vi "Main_Source.vi"() -> ()   [LabVIEW 2014]
panel:
  in  "Stop Button":bool
  out "error out":errorcluster
  in  "error in (no error)":errorcluster
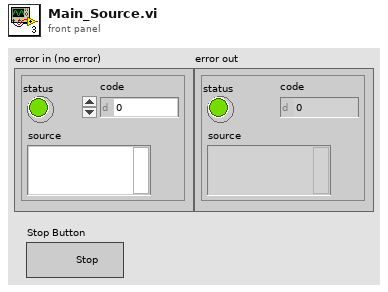
[diagram p1: front panel]
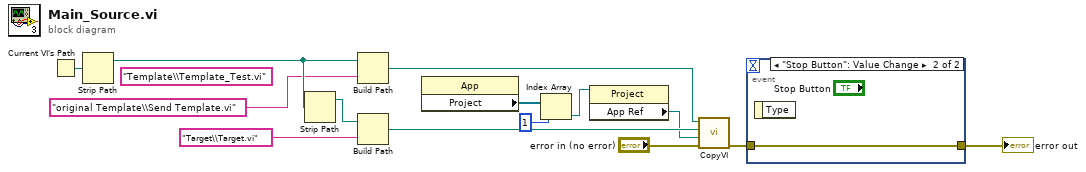
[diagram p0: block diagram]
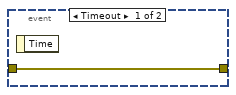
[diagram p2: hidden frame]
diagram:
  (unwired) "Template\\Template_Test.vi" ("name or relative path")
  n1 = Current VI's Path() -> (path=w13:path)
  n2 = Strip Path(path=w13) -> (stripped path=w7:path)  [unwired: 1 out]
  n3 = Strip Path(path=w7) -> (stripped path=w6:path)  [unwired: 1 out]
  n4 = Build Path(base path=w7, name or relative path="original Template\\Send Template.vi") -> (appended path=w12:path)
  n5 = Build Path(base path=w6, name or relative path="Target\\Target.vi") -> (appended path=w11:path)
  n6 = property class="App"() -> ("Project"=w5:refnum<vi>[])  [unwired: 2 in, 2 out]
  n7 = Index Array(array=w5, index=1) -> (element=w4:refnum<vi>)
  n8 = property class="Project"(reference=w4) -> ("App Ref"=w3:refnum<vi>)  [unwired: 1 in, 2 out]
  n9 = call "CopyVI.vi"("error in (no error)"="error in (no error)", "application reference (local)"=w3, "Empty File"=w11, "File to Copy"=w12) -> ("error out"=w9:errorcluster)  [unwired: 7 in]
  n10 = event shown="[1] \"Stop Button\": Value Change" {
    selector: _ -> [_ _]
    dyn-events: _ -> [_ _]
    timeout: _ -> [_ _]
    tunnel: w9 -> [w15 w16]
    tunnel: [w15 w16] -> w8
    event Timeout {
      n11 = event-data() -> ()  [unwired: 1 in, 1 out]
    }
    event "Stop Button": Value Change {
      n12 = event-data() -> ()  [unwired: 1 in, 1 out]
    }
  }
  "error out" <- w8
